vi "Configure Sweep (Step).vi"(0 "VISA resource name":refnum<visa-resource-name>, 1 "Step Spacing (0: Linear)":u16(ring) items=["Linear", "Logarithmic"], 2 "Number Of Points (2)":i32=2, 5 "Step Dwell (2 ms)":dbl=0.002, 7 "Frequency Start (100 kHz)":dbl=100000.0, 9 "Frequency Stop (100 kHz)":dbl=100000.0, 11 "error in (no error)":errorcluster, 12 "Power Start (-130 dB)":dbl=-130.0, 13 "Power Stop (-130 dB)":dbl=-130.0) -> (4 "VISA resource name out":refnum<visa-resource-name>, 15 "error out":errorcluster)   [LabVIEW 2018, in "Agilent PSG MXG Series.lvlib"]
doc: "Configures number of points, dwell time, start frequency, stop frequency, start amplitude and stop amplitude in the step sweep mode."
uses:
  Agilent PSG MXG Series.lvlib
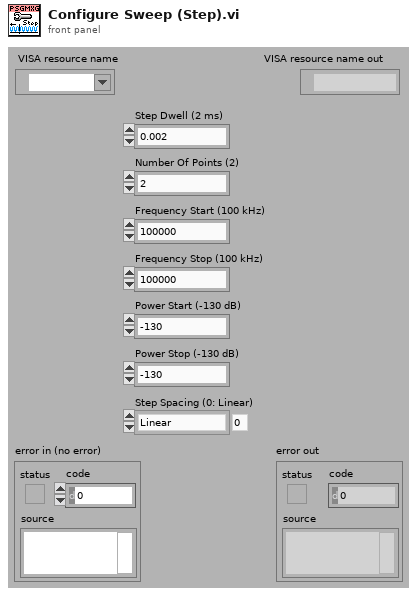
[diagram p1: front panel]
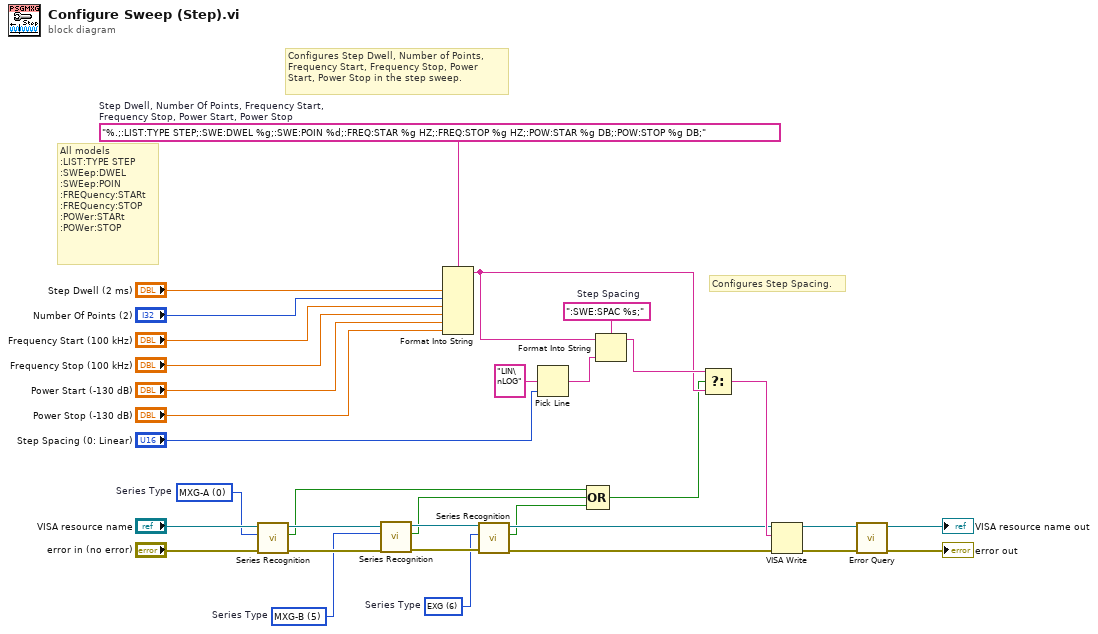
[diagram p0: block diagram]
diagram:
  w5 = u16 6 items=["MXG-A", "PSG", "PSG-A", "PSG-C", "PSG-D", "MXG-B", "EXG"]  # Series Type
  w10 = u16 5 items=["MXG-A", "PSG", "PSG-A", "PSG-C", "PSG-D", "MXG-B", "EXG"]  # Series Type
  w13 = u16 0 items=["MXG-A", "PSG", "PSG-A", "PSG-C", "PSG-D", "MXG-B", "EXG"]  # Series Type
  w26 = ":SWE:SPAC %s;"  # Step Spacing
  w33 = "%.;:LIST:TYPE STEP;:SWE:DWEL %g;:SWE:POIN %d;:FREQ:STAR %g HZ;:FREQ:STOP %g HZ;:POW:STAR %g DB;:POW:STOP %g DB;"  # Step Dwell, Number Of Points, Frequency Start, Frequency Stop, Power Start, Power Stop
  # "All models\n:LIST:TYPE STEP\n:SWEep:DWEL\n:SWEep:POIN\n:FREQuency:STARt\n:FREQuency:STOP\n:POWer:STARt\n:POWer:STOP"
  # "Configures Step Spacing."
  # "Configures Step Dwell, Number of Points,\nFrequency Start, Frequency Stop, Power\nStart, Power Stop in the step sweep."
  n1 = call "Series Recognition.vi"("error in (no error)"="error in (no error)", "Series Type (0: MXG)"=w13, "VISA resource name"="VISA resource name") -> ("error out"=w11:errorcluster, "Is Series Correct"=w4:bool, "VISA resource name out"=w12:refnum<visa-resource-name>)  [unwired: 1 in, 5 out]
  n2 = call "Series Recognition.vi"("error in (no error)"=w11, "Series Type (0: MXG)"=w10, "VISA resource name"=w12) -> ("error out"=w7:errorcluster, "Is Series Correct"=w3:bool, "VISA resource name out"=w9:refnum<visa-resource-name>)  [unwired: 1 in, 5 out]
  n3 = Format Into String(format string=w33, "Step Dwell (2 ms)", "Number Of Points (2)", "Frequency Start (100 kHz)", "Frequency Stop (100 kHz)", "Power Start (-130 dB)", "Power Stop (-130 dB)") -> (resulting string=w21:string)  [unwired: 2 in, 1 out]
  n4 = call "Series Recognition.vi"("error in (no error)"=w7, "Series Type (0: MXG)"=w5, "VISA resource name"=w9) -> ("error out"=w6:errorcluster, "Is Series Correct"=w2:bool, "VISA resource name out"=w8:refnum<visa-resource-name>)  [unwired: 1 in, 5 out]
  n5 = Pick Line(multi-line string="LIN\nLOG", line index="Step Spacing (0: Linear)") -> (output string=w25:string)  [unwired: 1 out]
  n6 = Compound Arithmetic op=OR(w4, w3, w2) -> (w1:bool)
  n7 = Format Into String(format string=w26, initial string=w21, w25) -> (resulting string=w22:string)  [unwired: 1 in, 1 out]
  n8 = Select(t=w22, s=w1, f=w21) -> (s? t:f=w20:string)
  n9 = VISA Write(VISA resource name=w8, write buffer=w20, error in (no error)=w6) -> (VISA resource name out=w19:refnum<visa-resource-name>, error out=w18:errorcluster)  [unwired: 1 out]
  n10 = call "Error Query.vi"("error in (no error)"=w18, "VISA resource name"=w19) -> ("error out"=→"error out":errorcluster, "VISA resource name out"=→"VISA resource name out":refnum<visa-resource-name>)  [unwired: 8 out]
